vi "RunPythonCode.vi"(6 "Path to Actuation Script":path=path "C:/Users/dpl/Documents/ob_egse/src/main.py", 7 "COM Port":i32=5 min=1 max=63 step=1, 8 "error in (no error)":errorcluster, 9 "TestPrefix":string="myfile", 11 "Output base directory":path=path "E:/LTM Tests/MechanismLTM") -> (0 "error out":errorcluster, 1 "return code":i32)   [LabVIEW 2025]
doc: "Run Python code to exercise Enfys ob_egse\n\ndpl@aber.ac.uk"
panel:
  out "command string":string
  out "standard error":string
  out "standard output":string
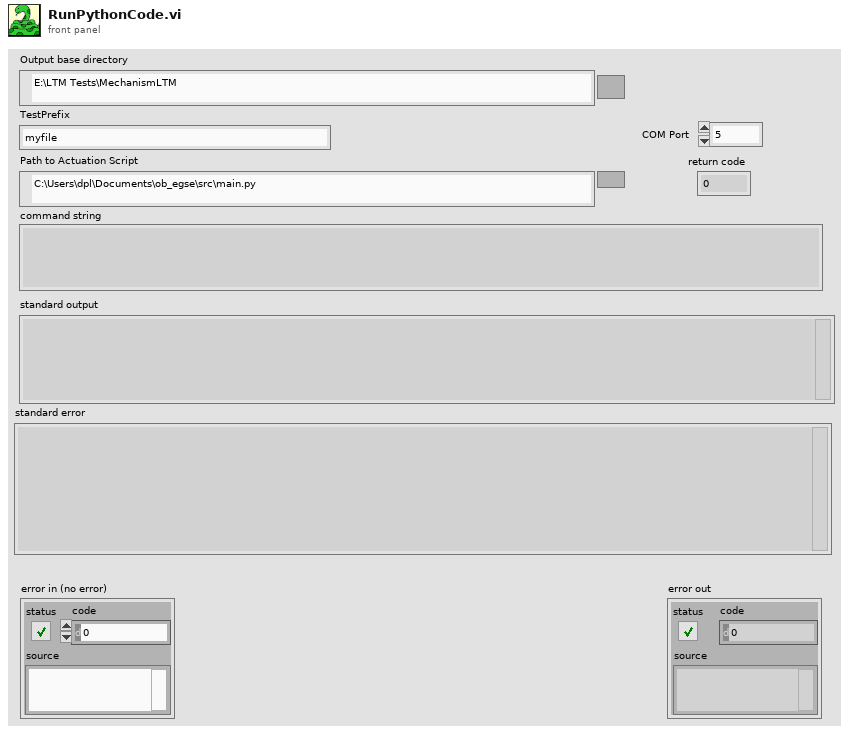
[diagram p1: front panel]
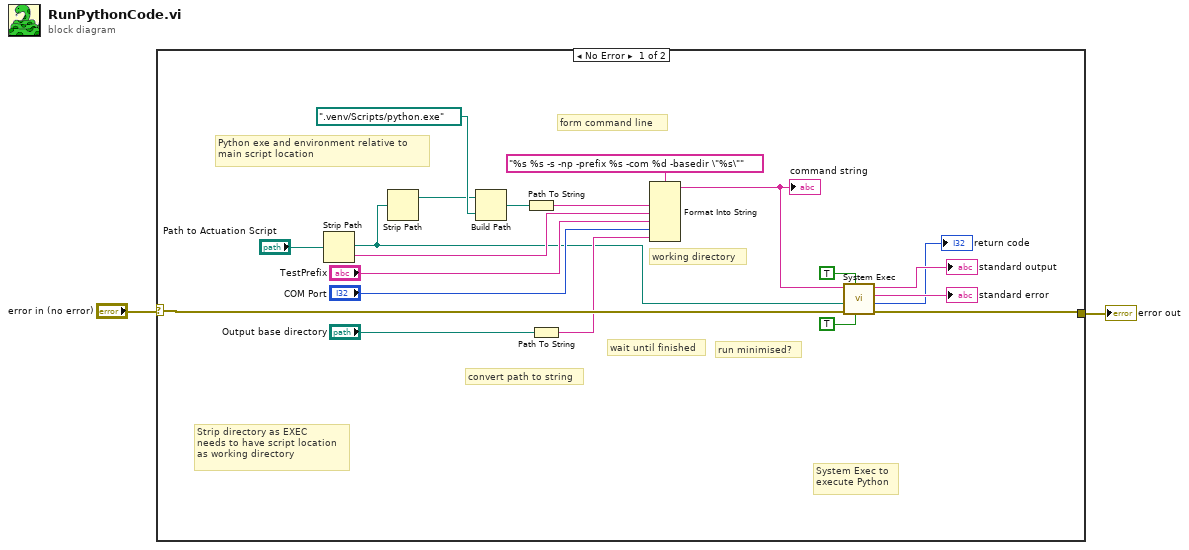
[diagram p0: block diagram]
diagram:
  n1 = case shown="No Error" "error in (no error)" {
    selector: "error in (no error)" -> [w15 w23]
    tunnel: [w6 w23] -> w1
    frame No Error {
      # "Python exe and environment relative to \nmain script location"
      # "convert path to string"
      # "working directory"
      # "Strip directory as EXEC\nneeds to have script location\nas working directory"
      # "run minimised?"
      # "wait until finished"
      # "System Exec to\nexecute Python"
      # "form command line"
      n2 = Strip Path(path="Path to Actuation Script") -> (stripped path=w5:path, name=w11:string)
      n3 = Strip Path(path=w5) -> (stripped path=w4:path)  [unwired: 1 out]
      n4 = Build Path(base path=w4, name or relative path=path ".venv/Scripts/python.exe") -> (appended path=w8:path)
      n5 = Path To String(path=w8) -> (string=w7:string)
      n6 = Path To String(path="Output base directory") -> (string=w14:string)
      n7 = Format Into String(format string="%s %s -s -np -prefix %s -com %d -basedir \"%s\"", w7, w11, "TestPrefix", "COM Port", w14) -> (resulting string=w18:string)  [unwired: 2 in, 1 out]
      "command string" <- w18
      n8 = call <vilib>:"System Exec.vi"("run minimized? (F)"=TRUE, "wait until completion? (T)"=TRUE, "error in (no error)"=w15, "working directory"=w5, "command line"=w18) -> ("error out"=w6:errorcluster, "return code"=→"return code":i32, "standard error"=→"standard error":string, "standard output"=→"standard output":string)  [unwired: 3 in]
    }
    frame Error {
    }
  }
  "error out" <- w1
